vi "Sort Fcurve metadata.vi"(0 "reference in":refnum<class "Fcurve.lvclass">, 5 "error in (no error)":errorcluster) -> (14 "reference out":refnum<class "Fcurve.lvclass">, 16 "Metadata out":T1, 19 "error out":errorcluster)   [LabVIEW 2019, in "Fcurve.lvclass"]
doc: "Sorts the Fcurve properties from the metadata input parameters"
uses:
  Fcurve.lvclass
  Metadata.ctl
  metadata_class/metadata.lvclass
panel:
  out "1/x":dbl
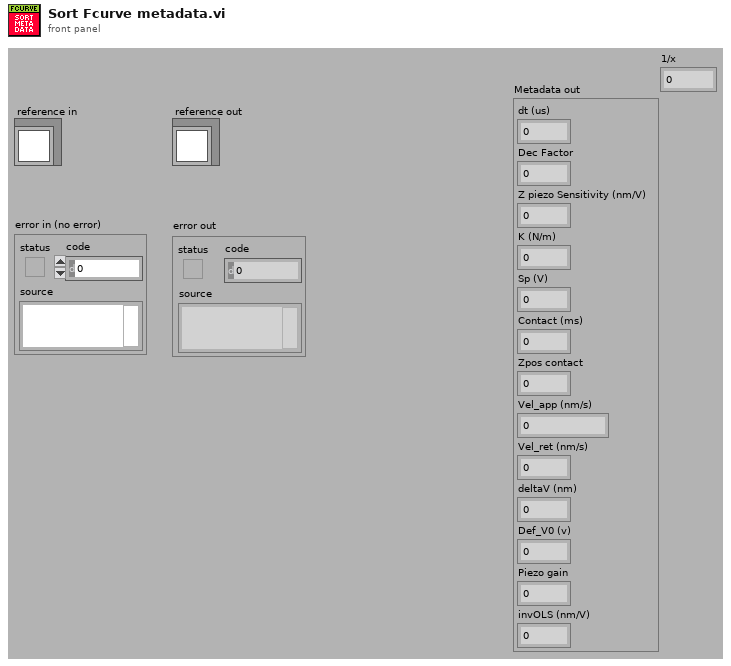
[diagram p1: front panel]
types:
  T1 = typedef "Fcurve.lvclass/Metadata.ctl" = cluster{"dt (us)":dbl, "Dec Factor":dbl, "Z piezo Sensitivity (nm/V)":dbl, "K (N/m)":dbl, "Sp (V)":dbl, "Contact (ms)":dbl, "Zpos contact":dbl, "Vel_app (nm/s)":dbl, "Vel_ret (nm/s)":dbl, "deltaV (nm)":dbl, "Def_V0 (v)":dbl, "Piezo gain":dbl, "invOLS (nm/V)":dbl}
  T2 = typedef "Fcurve.lvclass/ObjectAttributesRef.ctl" = refnum<data-value>
  T3 = typedef "Fcurve.lvclass/ObjectAttributes.ctl" = cluster{"MyAttribute":dbl, "Fcurve Metadata":T1, "Contact Spread of dev":dbl, "Tau Delay (ms)":dbl, "Points of contact":dbl, "Def_wfm":cluster{"Max":dbl, "Min":dbl}, "Zpos_wfm":cluster{"Max":dbl, "Min":dbl}, "Contact stat?":bool, "Real AI dt (s)":dbl, "Decimation":cluster{"App":cluster{"Dec":i32, "apply":bool}, "Con":cluster{"Dec":i32, "apply":bool}, "Ret":cluster{"Dec":i32, "apply":bool}}, "Segment def[0]":dbl, "Segment Zpos[0]":dbl, "Raw Datum":waveform(dbl)[], "Group metadata":T4, "M_data obj":refnum<class "metadata.lvclass">, "Channel name(s)":string[], "Segment fcurve data":cluster{"X":dbl[], "Y":dbl[]}[], "Segment duration":cluster{"Start":i32, "Duration":i32}[], "Segment info":T5[], "Segment durations (S)":dbl[], "Segments Maxmin":T7[]}
  T4 = typedef "TDMS_DataHandler.lvclass/Fcurve Meta data.ctl" = cluster{"property names":string[], "property values":variant[]}
  T5 = typedef "Fcurve.lvclass/Fcurve segments --cluster.ctl" = cluster{"type":T6, "nb points":i32, "dec factor":u32, "sampling rate (S/s)":u32}
  T6 = typedef "metadata.lvclass/Segment type--combobox.ctl" = string
  T7 = typedef "Fcurve.lvclass/Segment MaxMin --cluster.ctl" = cluster{"Def":cluster{"max value":dbl, "min value":dbl}, "Zpos":cluster{"max value":dbl, "min value":dbl}}
  T8 = typedef "metadata.lvclass/Fcurve segment.ctl" = cluster{"type":T6, "fast_fpga_trigger":bool, "nb":u8, "duration (ticks)":i64, "nb points":i32, "sampling rate (S/s)":u32, "Zpiezo control out":string, "initial deflection (V)":dbl, "relative setpoint":bool, "setpoint on":bool, "setpoint (V)":dbl, "setpoint trigger channel":string, "velocity (V/tick)":dbl, "Z position setpoint trigger (V)":dbl, "Z retract length (V)":dbl, "dec factor":u32}
  T9 = typedef "metadata.lvclass/XYZ piezos parameters.ctl" = cluster{"X stage piezo sensitivity (nm/V)":dbl, "X stage piezo gain":dbl, "X velocity (V/tick)":dbl, "X closed loop":bool, "Y stage piezo sensitivity (nm/V)":dbl, "Y stage piezo gain":dbl, "Y velocity (V/tick)":dbl, "Y closed loop":bool, "Z stage piezo sensitivity (nm/V)":dbl, "Z stage piezo gain":dbl, "Z closed loop":bool, "X position (V)":dbl, "Y position (V)":dbl}
  T10 = typedef "metadata.lvclass/Cantilever info parameters.ctl" = cluster{"spring constant calib method":string, "invOLS calib method":string, "thermal calib deflection channel":string, "model":string, "shape":string, "tip geometry":string, "Laser sum (V)":dbl, "Laser power (mA)":dbl, "invOLS_(nm/V)":dbl, "spring constant nominal (N/m)":dbl, "spring constant calib (N/m)":dbl, "resosnance frequency air calib (Hz)":dbl, "resosnance frequency calib (Hz)":dbl, "quality factor":dbl, "Acoefficident_GCI_(nN.s^1.3/m)":dbl, "half angle (deg)":dbl, "tip radius (m)":dbl, "tip height (m)":dbl, "system mount angle (deg)":dbl}
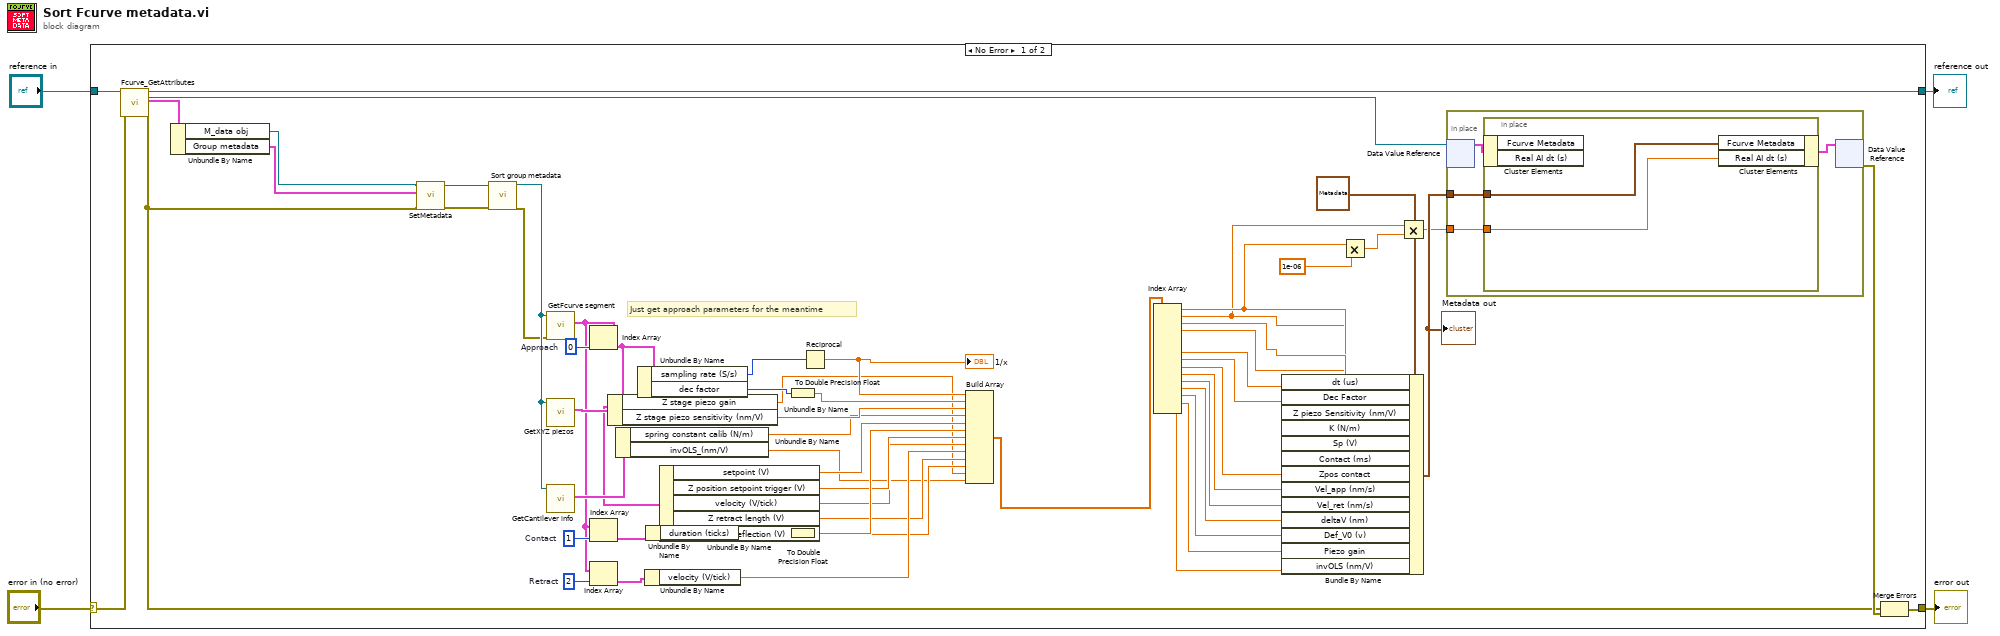
[diagram p0: block diagram]
diagram:
  n1 = case shown="No Error" "error in (no error)" {
    selector: "error in (no error)" -> [w62 w70]
    tunnel: [w57 w70] -> w3
    tunnel: [w61 w69] -> w1
    tunnel: "reference in" -> [w59 w69]
    frame No Error {
      w18 = 2  # Retract
      w20 = 0  # Approach
      w24 = 1  # Contact
      # "Just get approach parameters for the meantime"
      n2 = call "Fcurve_GetAttributes.vi"("reference in"=w59, "error in (no error)"=w62) -> ("reference out"=w61:refnum<class "Fcurve.lvclass">, "attributes ref"=w56:T2, "attributes"=w60:T3, "error out"=w7:errorcluster)  [unwired: 14 in]
      n3 = Unbundle By Name(w60) -> ("M_data obj"=w9:refnum<class "metadata.lvclass">, "Group metadata"=w5:T4)
      n4 = call-dynamic "SetMetadata.vi"("error in (no error)"=w7, "Metadata"=w5, "reference in"=w9) -> ("error out"=w6:errorcluster, "reference out"=w8:refnum<class "metadata.lvclass">)  [unwired: 7 in]
      n5 = call-dynamic "Sort group metadata.vi"("reference in"=w8, "error in (no error)"=w6) -> ("reference out"=w36:refnum<class "metadata.lvclass">, "error out"=w35:errorcluster)  [unwired: 16 in]
      n6 = call-dynamic "GetFcurve segment.vi"("error in (no error)"=w35, "reference in"=w36) -> ("Fcurve segment"=w19:T8[])  [unwired: 7 in, 2 out]
      n7 = call-dynamic "GetXYZ piezos.vi"("reference in"=w36) -> ("XYZ piezos"=w31:T9)  [unwired: 8 in, 2 out]
      n8 = call-dynamic "GetCantilever info.vi"("reference in"=w36) -> ("Cantilever info"=w30:T10)  [unwired: 8 in, 2 out]
      n9 = Index Array(array=w19, index=w20) -> (element=w26:T8)
      n10 = Index Array(array=w19, index=w24) -> (element=w23:T8)
      n11 = Index Array(array=w19, index=w18) -> (element=w15:T8)
      n12 = Unbundle By Name(w31) -> ("Z stage piezo gain"=w11:dbl, "Z stage piezo sensitivity (nm/V)"=w28:dbl)
      n13 = Unbundle By Name(w30) -> ("spring constant calib (N/m)"=w27:dbl, "invOLS_(nm/V)"=w10:dbl)
      n14 = Unbundle By Name(w26) -> ("sampling rate (S/s)"=w34:u32, "dec factor"=w32:u32)
      n15 = Unbundle By Name(w15) -> ("velocity (V/tick)"=w14:dbl)
      n16 = Unbundle By Name(w23) -> ("duration (ticks)"=w22:i64)
      n17 = Unbundle By Name(w26) -> ("setpoint (V)"=w25:dbl, "Z position setpoint trigger (V)"=w17:dbl, "velocity (V/tick)"=w16:dbl, "Z retract length (V)"=w13:dbl, "initial deflection (V)"=w12:dbl)
      n18 = To Double Precision Float(number=w32) -> (double precision float=w29:dbl)
      n19 = To Double Precision Float(number=w22) -> (double precision float=w21:dbl)
      n20 = Reciprocal(x=w34) -> (1/x=w33:dbl)
      "1/x" <- w33
      n21 = Build Array(w33, w29, w28, w27, w25, w21, w17, w16, w14, w13, w12, w11, w10) -> (w53:dbl[])
      n22 = Index Array(array=w53) -> (element #1=w39:dbl, element #2=w37:dbl, element #3=w52:dbl, element #4=w51:dbl, element #5=w50:dbl, element #6=w49:dbl, element #7=w48:dbl, element #8=w47:dbl, element #9=w46:dbl, element #10=w45:dbl, element #11=w44:dbl, element #12=w43:dbl, element #13=w42:dbl)  [unwired: 13 in]
      n23 = Bundle By Name(cluster=T1 {"dt (us)"=0.0, "Dec Factor"=0.0, "Z piezo Sensitivity (nm/V)"=0.0, "K (N/m)"=0.0, "Sp (V)"=0.0, "Contact (ms)"=0.0, "Zpos contact"=0.0, "Vel_app (nm/s)"=0.0, "Vel_ret (nm/s)"=0.0, "deltaV (nm)"=0.0, "Def_V0 (v)"=0.0, "Piezo gain"=0.0, "invOLS (nm/V)"=0.0} ("Fcurve Metadata"), "dt (us)"=w39, "Dec Factor"=w37, "Z piezo Sensitivity (nm/V)"=w52, "K (N/m)"=w51, "Sp (V)"=w50, "Contact (ms)"=w49, "Zpos contact"=w48, "Vel_app (nm/s)"=w47, "Vel_ret (nm/s)"=w46, "deltaV (nm)"=w45, "Def_V0 (v)"=w44, "Piezo gain"=w43, "invOLS (nm/V)"=w42) -> (w54:T1)
      "Metadata out" <- w54
      n24 = Multiply(x=w39, y=1e-06) -> (x*y=w40:dbl)
      n25 = Multiply(x=w37, y=w40) -> (x*y=w38:dbl)
      n26 = in-place {
        in-place-border: w54 -> [w64]
        in-place-border: w38 -> [w63]
        n27 = in-place-dvr #1(w56) -> (w65:T3)  [unwired: 1 out]
        n28 = in-place {
          in-place-border: w64 -> [w68]
          in-place-border: w63 -> [w67]
          n29 = in-place-cluster #2(w65) -> ()  [unwired: 2 out]
          n30 = in-place-cluster #2("Fcurve Metadata"=w68, "Real AI dt (s)"=w67) -> (w66:T3)
        }
        n31 = in-place-dvr #1(w66) -> (w58:errorcluster)  [unwired: 1 out]
      }
      n32 = Merge Errors(w7, w58) -> (w57:errorcluster)
    }
    frame Error {
    }
  }
  "error out" <- w3
  "reference out" <- w1
